vi "SVX Convert Colormap to Waterfall.vi"(8 "error in (no error)":errorcluster, 11 "colormap":T2) -> (0 "error out":errorcluster, 1 "y-axis unit label":string, 2 "x-axis unit label":string, 3 "waterfall graph data out":T1, 4 "z-axis unit label":string)   [LabVIEW 2017, in "SoundVib_SpectralDisplay.lvlib"]
doc: "Converts Colormap data to Waterfall Graph data."
uses:
  <vilib>/addons/Sound and Vibration/Order Analysis/Data Presentation/SoundVib_SpectralDisplay.lvlib
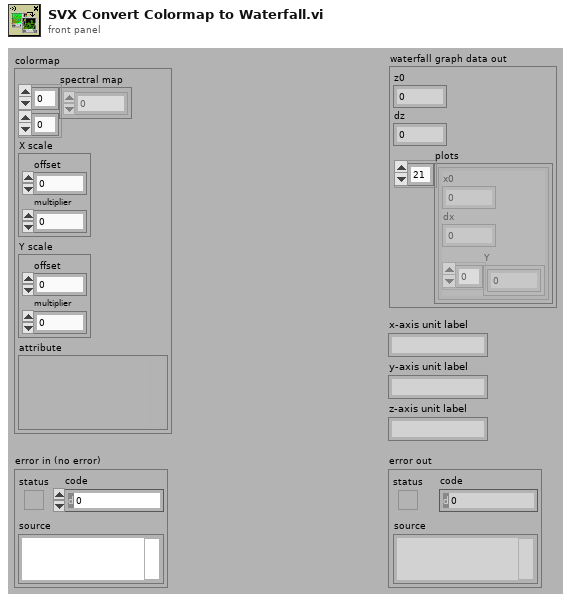
[diagram p1: front panel]
types:
  T1 = cluster{"z0":dbl, "dz":dbl, "plots":cluster{"x0":dbl, "dx":dbl, "Y":dbl[]}[]}
  T2 = cluster{"spectral map":dbl[][], "X scale":cluster{"offset":dbl, "multiplier":dbl}, "Y scale":cluster{"offset":dbl, "multiplier":dbl}, "attribute":variant}
  T3 = cluster{"z0":dbl, "dz":dbl, "Plots":cluster{"x0":dbl, "dx":dbl, "Y":dbl[]}[]}
  T4 = enum16{"Frequency-Time", "Time-Frequency", "Order-Time", "Time-Order", "Frequency-RPM", "RPM-Frequency", "Order-RPM", "RPM-Order"}
  T5 = cluster{"offset":dbl, "multiplier":dbl, "spectral map":dbl[]}
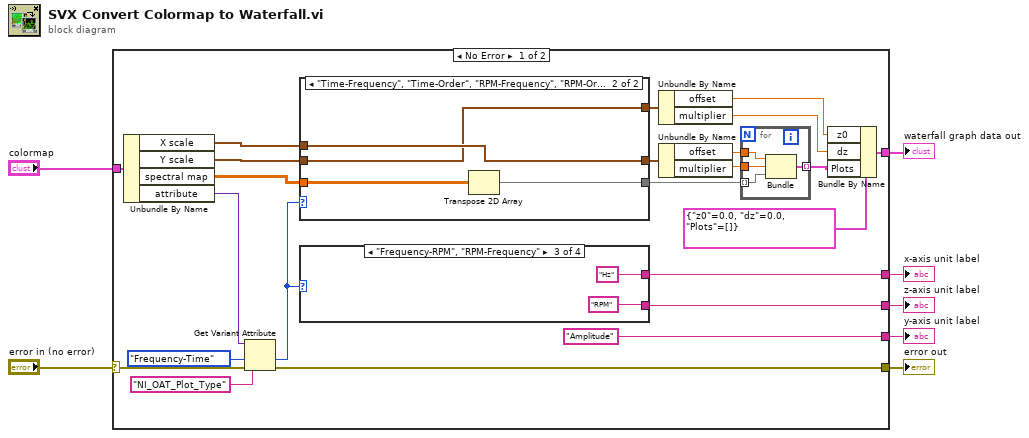
[diagram p0: block diagram]
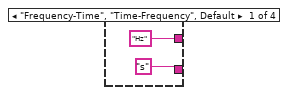
[diagram p2: hidden frame]
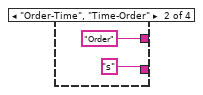
[diagram p3: hidden frame]
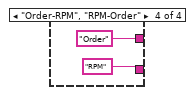
[diagram p4: hidden frame]
diagram:
  n1 = case shown="No Error" "error in (no error)" {
    selector: "error in (no error)" -> [w9 w50]
    tunnel: "colormap" -> [w28 _]
    tunnel: [w22 _] -> w6
    tunnel: [w14 _] -> w5
    tunnel: [w13 _] -> w4
    tunnel: ["Amplitude" ("Z axis unit label") _] -> w3
    tunnel: [w11 w50] -> w2
    frame No Error {
      n2 = Unbundle By Name(w28) -> ("X scale"=w20:cluster{"offset":dbl, "multiplier":dbl}, "Y scale"=w19:cluster{"offset":dbl, "multiplier":dbl}, "spectral map"=w27:dbl[][], "attribute"=w10:variant)
      n3 = Get Variant Attribute(Variant=w10, name="NI_OAT_Plot_Type", default value (empty Variant)=T4."Frequency-Time" ("plot type 2"), error in=w9) -> (value=w15:T4, error out=w11:errorcluster)  [unwired: 2 out]
      n4 = case shown="\"Time-Frequency\", \"Time-Order\", \"RPM-Frequency\", \"RPM-Order\"" w15 {
        tunnel: w27 -> [w39 w45]
        tunnel: [w39 w44] -> w21
        tunnel: w20 -> [w41 w43]
        tunnel: [w40 w43] -> w17
        tunnel: w19 -> [w40 w42]
        tunnel: [w41 w42] -> w18
        frame "Frequency-Time", "Order-Time", "Frequency-RPM", "Order-RPM", Default {
        }
        frame "Time-Frequency", "Time-Order", "RPM-Frequency", "RPM-Order" {
          n5 = Transpose 2D Array(2D array=w45) -> (transposed array=w44:dbl[][])
        }
      }
      n6 = case shown="\"Frequency-RPM\", \"RPM-Frequency\"" w15 {
        tunnel: ["Hz" ("name") "Order" ("name") "Hz" ("name") "Order" ("name")] -> w14
        tunnel: ["s" ("name") "s" ("name") "RPM" ("name") "RPM" ("name")] -> w13
        frame "Frequency-Time", "Time-Frequency", Default {
        }
        frame "Order-Time", "Time-Order" {
        }
        frame "Frequency-RPM", "RPM-Frequency" {
        }
        frame "Order-RPM", "RPM-Order" {
        }
      }
      n7 = Unbundle By Name(w18) -> ("offset"=w8:dbl, "multiplier"=w23:dbl)
      n8 = Unbundle By Name(w17) -> ("offset"=w26:dbl, "multiplier"=w25:dbl)
      n9 = for {
        tunnel: w21 -> [w49] mode=indexing
        tunnel: w26 -> [w48]
        tunnel: w25 -> [w47]
        tunnel: [w46] -> w16 mode=indexing
        n10 = Bundle("offset"=w48, "multiplier"=w47, "spectral map"=w49) -> (w46:T5)  [unwired: 1 in]
      }
      n11 = Bundle By Name(cluster=T3 {"z0"=0.0, "dz"=0.0, "Plots"=[]} ("Waterfall Graph"), "z0"=w8, "dz"=w23, "Plots"=w16) -> (w22:T3)
    }
    frame Error {
    }
  }
  "waterfall graph data out" <- w6
  "x-axis unit label" <- w5
  "z-axis unit label" <- w4
  "y-axis unit label" <- w3
  "error out" <- w2
